vi "Online_Target.vi"() -> ()   [LabVIEW 2021]
uses:
  Model_Updating_Classes/DROPBEAR_Model_Updating/DROPBEAR_Model_Updating.lvclass
  Model_Updating_Classes/MOCKBEAR/MOCKBEAR.lvclass
panel:
  out "Process_Start":bool
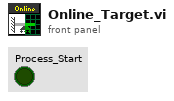
[diagram p1: front panel]
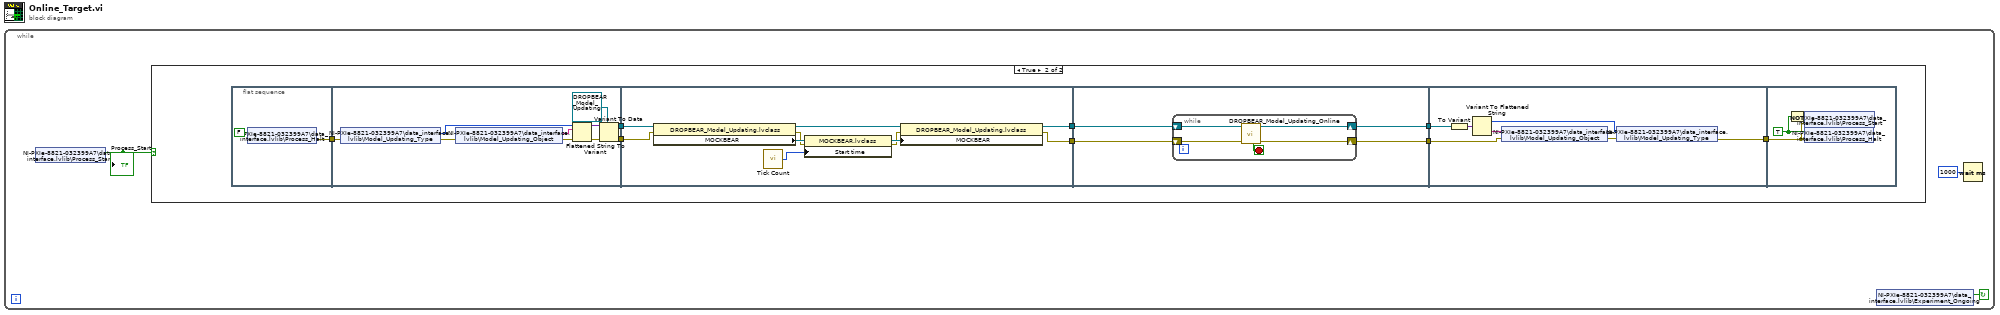
[diagram p0: block diagram]
diagram:
  n1 = while {
    stop <- w2 continue-if-true
    n2 = shared-variable "NI-PXIe-8821-032399A7\\data_interface.lvlib\\Process_Start"() -> (w3:bool)  [unwired: 1 in, 1 out]
    "Process_Start" <- w3
    n3 = case shown="True" w3 {
      frame False {
      }
      frame True {
        n4 = flat-sequence {
          tunnel: [w12] -> w11
          tunnel: [w16] -> w10
          tunnel: [w17] -> w9
          tunnel: w11 -> [w14]
          tunnel: w10 -> [w24]
          tunnel: [w27] -> w8
          tunnel: w9 -> [w28]
          tunnel: [w26] -> w7
          tunnel: w8 -> [w37]
          tunnel: [w36] -> w6
          tunnel: w7 -> [w35]
          tunnel: [w34] -> w5
          tunnel: w6 -> [w49]
          tunnel: w5 -> [w44]
          tunnel: [w43] -> w4
          tunnel: w4 -> [w50]
          frame #0 {
            n5 = shared-variable "NI-PXIe-8821-032399A7\\data_interface.lvlib\\Process_Halt"(FALSE ("Process_Halt")) -> (error out=w12:errorcluster)  [unwired: 1 in]
          }
          frame #1 {
            n6 = shared-variable "NI-PXIe-8821-032399A7\\data_interface.lvlib\\Model_Updating_Type"(error in=w14) -> (w21:i16[], error out=w18:errorcluster)
            n7 = shared-variable "NI-PXIe-8821-032399A7\\data_interface.lvlib\\Model_Updating_Object"(error in=w18) -> (w20:string, error out=w19:errorcluster)
            n8 = Flattened String To Variant(4:w19, 6:w20, 7:w21) -> (0:w23:errorcluster, 3:w22:variant)
            n9 = Variant To Data(error in=w23, type=refnum<class "DROPBEAR_Model_Updating.lvclass"> refnum ("DROPBEAR_Model_Updating.lvclass"), Variant=w22) -> (data=w16:refnum<class "DROPBEAR_Model_Updating.lvclass">, error out=w17:errorcluster)
          }
          frame #2 {
            n10 = property class="DROPBEAR_Model_Updating.lvclass"(reference=w24, error in=w28) -> (reference out=w31:refnum<class "DROPBEAR_Model_Updating.lvclass">, error out=w25:errorcluster, "MOCKBEAR"=w33:refnum<class "MOCKBEAR.lvclass">)
            n11 = call "Tick Count"() -> ("Tick Count(uSec)"=w30:u32)
            n12 = property class="MOCKBEAR.lvclass"(reference=w33, error in=w25, "Start time"=w30) -> (reference out=w32:refnum<class "MOCKBEAR.lvclass">, error out=w29:errorcluster)
            n13 = property class="DROPBEAR_Model_Updating.lvclass"(reference=w31, error in=w29, "MOCKBEAR"=w32) -> (reference out=w27:refnum<class "DROPBEAR_Model_Updating.lvclass">, error out=w26:errorcluster)
          }
          frame #3 {
            n14 = while {
              shift-right: [w40] -> w36
              shift-left: w37 -> [w42]
              shift-right: [w39] -> w34
              shift-left: w35 -> [w41]
              stop <- w38 stop-if-true
              n15 = call-dynamic "DROPBEAR_Model_Updating_Online.vi"("error in (no error)"=w41, "DROPBEAR_Model_Updating in"=w42) -> ("error out"=w39:errorcluster, "DROPBEAR_Model_Updating out"=w40:refnum<class "DROPBEAR_Model_Updating.lvclass">, "looping"=w38:bool)  [unwired: 7 in]
            }
          }
          frame #4 {
            n16 = To Variant(anything=w49) -> (Variant=w45:variant)
            n17 = Variant To Flattened String(Variant=w45) -> (data string=w48:string, 1:w46:i16[])
            n18 = shared-variable "NI-PXIe-8821-032399A7\\data_interface.lvlib\\Model_Updating_Object"(w48, error in=w44) -> (error out=w47:errorcluster)
            n19 = shared-variable "NI-PXIe-8821-032399A7\\data_interface.lvlib\\Model_Updating_Type"(w46, error in=w47) -> (error out=w43:errorcluster)
          }
          frame #5 {
            w52 = TRUE ("Process_Halt")
            n20 = Not(x=w52) -> (.not. x?=w51:bool)
            n21 = shared-variable "NI-PXIe-8821-032399A7\\data_interface.lvlib\\Process_Start"(w51, error in=w50) -> ()  [unwired: 1 out]
            n22 = shared-variable "NI-PXIe-8821-032399A7\\data_interface.lvlib\\Process_Halt"(w52, error in=w50) -> ()  [unwired: 1 out]
          }
        }
      }
    }
    n23 = shared-variable "NI-PXIe-8821-032399A7\\data_interface.lvlib\\Experiment_Ongoing"() -> (w2:bool)  [unwired: 1 in, 1 out]
    n24 = Wait (ms)(milliseconds to wait=u32 1000) -> ()  [unwired: 1 out]
  }
